vi "4.7.vi"() -> ()   [LabVIEW 2017]
panel:
  out "随机数":i32
  out "输入值":i32
  out "猜的次数":i32
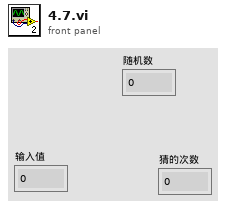
[diagram p1: front panel]
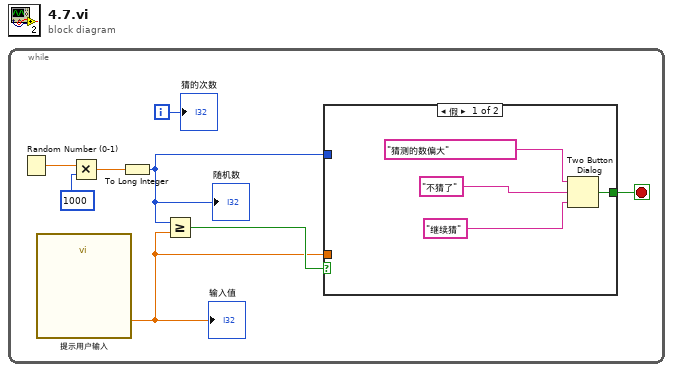
[diagram p0: block diagram]
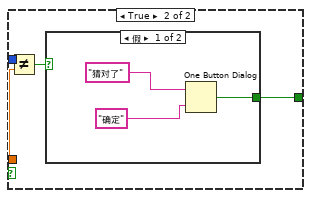
[diagram p2: hidden frame]
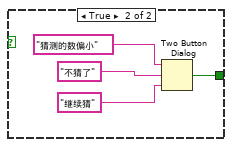
[diagram p3: hidden frame]
diagram:
  n1 = while {
    i -> [w5]
    stop <- w6 stop-if-true
    n2 = Random Number (0-1)() -> (number: 0 to 1=w8:dbl)
    n3 = call "提示用户输入"() -> ("请在1-1000猜"=w3:dbl)  [unwired: 17 in, 2 out]
    "输入值" <- w3
    n4 = Multiply(x=w8, y=1000) -> (x*y=w2:dbl)
    n5 = To Long Integer(number=w2) -> (32bit integer=w1:i32)
    "随机数" <- w1
    n6 = Greater Or Equal?(x=w1, y=w3) -> (x >= y?=w4:bool)
    n7 = case shown="假" w4 {
      tunnel: w3 -> [_ w13]
      tunnel: w1 -> [_ w14]
      tunnel: [w11 w16] -> w6
      frame False {
        n8 = Two Button Dialog(message="猜测的数偏大", 1:"继续猜", 2:"不猜了") -> (T button?=w11:bool)
      }
      frame True {
        n9 = Not Equal?(x=w14, y=w13) -> (x != y?=w15:bool)
        n10 = case shown="假" w15 {
          tunnel: [w17 w22] -> w16
          frame False {
            n11 = One Button Dialog(message="猜对了", button name ("OK")="确定") -> (true=w17:bool)
          }
          frame True {
            n12 = Two Button Dialog(message="猜测的数偏小", 1:"继续猜", 2:"不猜了") -> (T button?=w22:bool)
          }
        }
      }
    }
    "猜的次数" <- w5
  }
